vi "Test.Maui 2.0.Initialize.Plenty.Subpanels.Subpanel 1.vi"(8 "error in":errorcluster) -> (0 "error out":errorcluster)   [LabVIEW 2020]
uses:
  Maui 2.0/Maui 2.0.lvclass
  C:/Program Files (x86)/National Instruments/LabVIEW 2020/vi.lib/JKI/JKI SMO/SMO/SMO.lvclass
  Helper/Test Helper 1/Test Helper 1.lvclass
  <vilib>/addons/_JKI Toolkits/Caraya/classes/Assert/Assert Equal Value_Variant.vi
  <vilib>/JKI/JKI SMO/SMO/SMO.lvclass
  <vilib>/addons/_JKI Toolkits/Caraya/classes/Test/Test.lvclass
  <vilib>/addons/_JKI Toolkits/Caraya/classes/Assert/Assert.lvclass
panel:
  in  "Ring 2":u16(ring) items=["Test Helper 1", "Test Helper 1", "Maui 2.0", "None"]
  in  "Ring":u16(ring) items=["Test Helper 1", "Test Helper 1", "Maui 2.0", "None"]
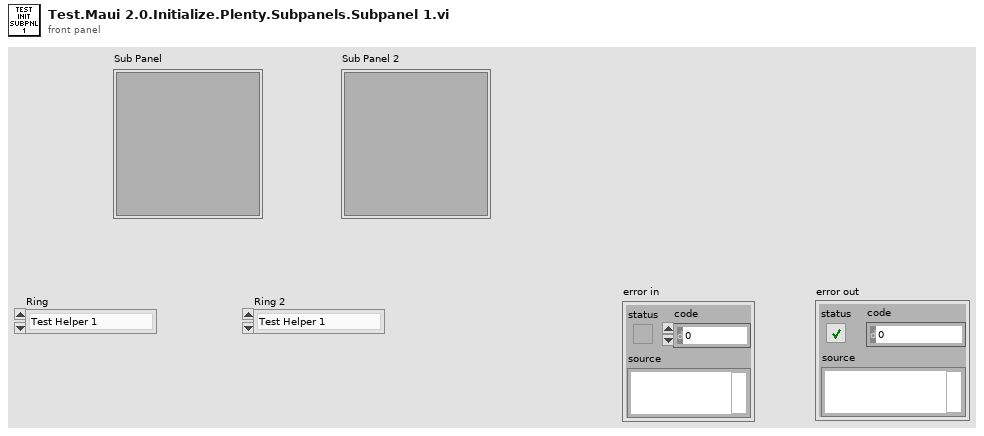
[diagram p1: front panel]
types:
  T1 = cluster{"Ring":refnum<vi>, "Sub Panel":refnum<vi>}
  T2 = cluster{"Ring 2":refnum<vi>, "Sub Panel 2":refnum<vi>}
  T3 = cluster{"Ring 2":refnum<vi>, "Sub Panel 2":refnum<vi>}[]
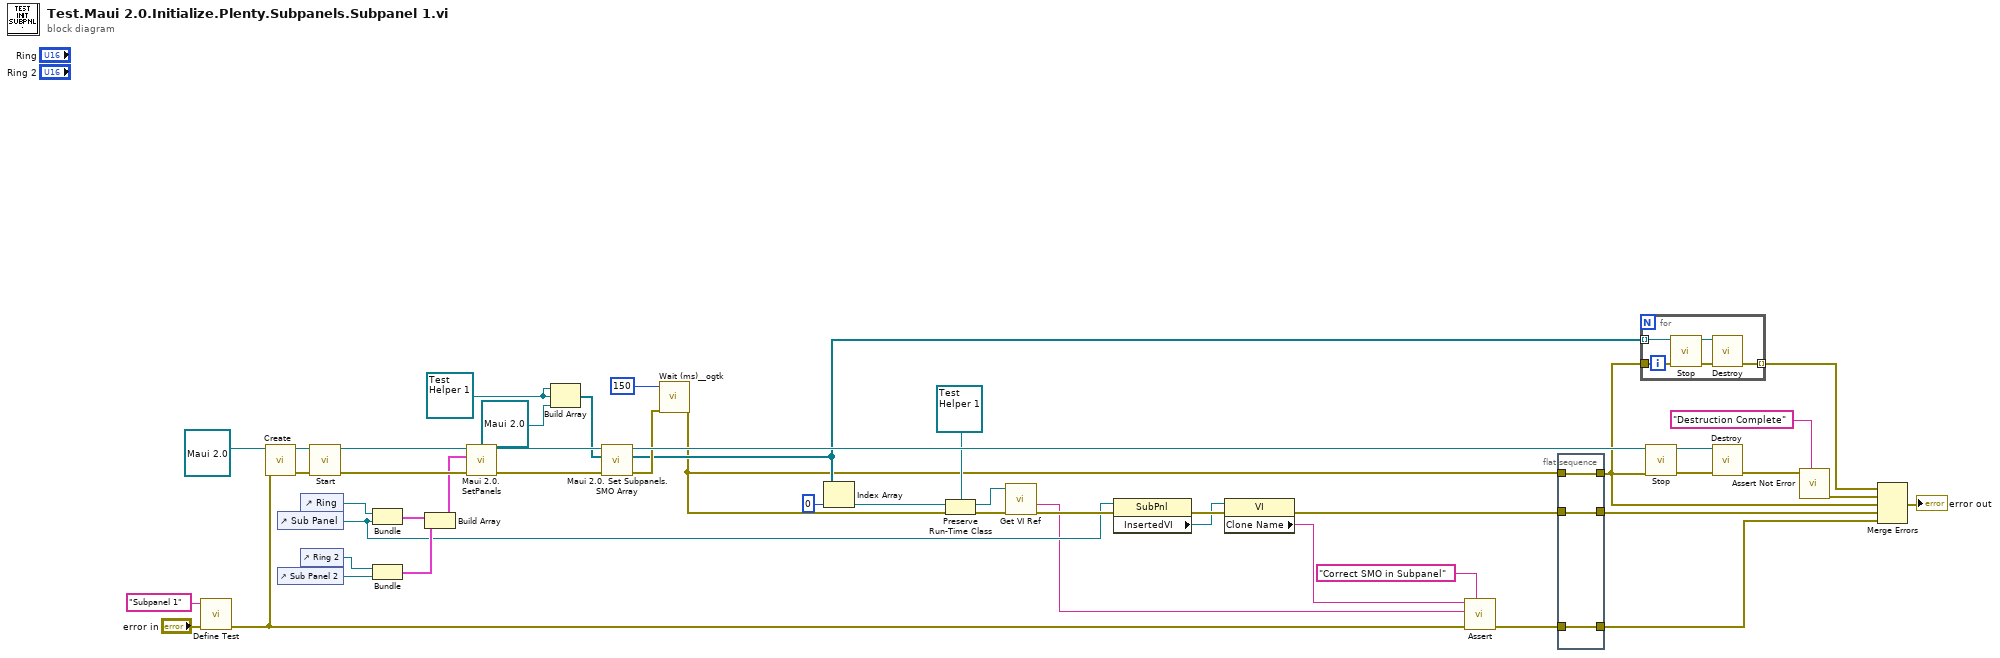
[diagram p0: block diagram]
diagram:
  w17 = refnum<class "Test Helper 1.lvclass"> refnum ("Test Helper 1.lvclass")
  n1 = call <vilib>:"Define Test.vi"("error in (no error)"="error in", "Label (VI Title)"="Subpanel 1") -> ("error out"=w20:errorcluster)  [unwired: 9 in]
  n2 = call <vilib>:"Create.vi"("error in (no error)"=w20, "SMO"=refnum<class "Maui 2.0.lvclass"> refnum ("Maui 2.0 in")) -> ("error out"=w48:errorcluster, "SMO out"=w41:refnum<class "Maui 2.0.lvclass">)  [unwired: 7 in, 1 out]
  n3 = control-ref of="Sub Panel"() -> (w9:refnum<vi>)
  n4 = control-ref of="Sub Panel 2"() -> (w44:refnum<vi>)
  n5 = control-ref of="Ring"() -> (w34:refnum<vi>)
  n6 = control-ref of="Ring 2"() -> (w45:refnum<vi>)
  n7 = call <vilib>:"Start.vi"("error in (no error)"=w48, "SMO"=w41) -> ("error out"=w47:errorcluster, "SMO out"=w39:refnum<class "Maui 2.0.lvclass">)  [unwired: 8 in]
  n8 = Bundle("Ring"=w34, "Sub Panel"=w9) -> (w43:T1)  [unwired: 1 in]
  n9 = Bundle("Ring 2"=w45, "Sub Panel 2"=w44) -> (w42:T2)  [unwired: 1 in]
  n10 = Build Array(w43, w42) -> (w35:T3)
  n11 = call "Maui 2.0.SetPanels.vi"("error in (no error)"=w47, "Set Panels"=w35, "Maui 2.0"=w39) -> ("error out"=w46:errorcluster, "Maui 2.0 out"=w38:refnum<class "Maui 2.0.lvclass">)  [unwired: 7 in]
  n12 = Build Array(w17, w17, refnum<class "Maui 2.0.lvclass"> refnum ("Maui 2.0 in")) -> (w36:refnum<class "SMO.lvclass">[])
  n13 = call-dynamic "Maui 2.0. Set Subpanels.SMO Array.vi"("error in (no error)"=w46, "Subpanels in"=w36, "Maui 2.0 in"=w38) -> ("error out"=w23:errorcluster, "Subpanels Out"=w5:refnum<class "SMO.lvclass">[], "Maui 2.0 out"=w31:refnum<class "Maui 2.0.lvclass">)  [unwired: 6 in]
  n14 = call <userlib>:"Wait (ms)__ogtk.vi"("error in (no error)"=w23, "milliseconds to wait"=u32 150) -> ("error out"=w4:errorcluster)  [unwired: 8 in, 1 out]
  n15 = Index Array(array=w5, index=0) -> (element=w19:refnum<class "SMO.lvclass">)
  n16 = Preserve Run-Time Class(object in=w19, error in=w4, 2:refnum<class "Test Helper 1.lvclass"> refnum ("Test Helper 1.lvclass")) -> (object out=w16:refnum<class "Test Helper 1.lvclass">, error out=w15:errorcluster)
  n17 = call-dynamic "Get VI Ref.vi"("error in (no error)"=w15, "Test Helper 1 in"=w16) -> ("error out"=w14:errorcluster, "VI Clone Name"=w3:string)  [unwired: 6 in, 2 out]
  n18 = property on="Property Node" class="SubPnl"(reference=w9, error in=w14) -> (error out=w12:errorcluster, "InsertedVI"=w10:refnum<vi>)  [unwired: 1 out]
  n19 = property on="Property Node" class="VI"(reference=w10, error in=w12) -> (error out=w11:errorcluster, "Clone Name"=w7:string)  [unwired: 1 out]
  n20 = call-poly <vilib>:"Assert.vi"("Label"="Correct SMO in Subpanel", "error in (no error)"=w20, "Y"=w3, "X"=w7) -> ("error out"=w8:errorcluster)  [unwired: 7 in]
  n21 = flat-sequence {
    tunnel: w4 -> [w51]
    tunnel: w11 -> [w50]
    tunnel: w8 -> [w49]
    tunnel: [w51] -> w21
    tunnel: [w50] -> w25
    tunnel: [w49] -> w24
    frame #0 {
    }
  }
  n22 = for {
    tunnel: w5 -> [w55] mode=indexing
    tunnel: w21 -> [w54]
    tunnel: [w52] -> w22 mode=indexing
    n23 = call <vilib>:"Stop.vi"("error in (no error)"=w54, "SMO"=w55) -> ("error out"=w53:errorcluster, "SMO out"=w56:refnum<class "SMO.lvclass">)  [unwired: 8 in]
    n24 = call <vilib>:"Destroy.vi"("error in (no error)"=w53, "SMO"=w56) -> ("error out"=w52:errorcluster)  [unwired: 9 in]
  }
  n25 = call <vilib>:"Stop.vi"("error in (no error)"=w21, "SMO"=w31) -> ("error out"=w29:errorcluster, "SMO out"=w30:refnum<class "Maui 2.0.lvclass">)  [unwired: 8 in]
  n26 = call <vilib>:"Destroy.vi"("error in (no error)"=w29, "SMO"=w30) -> ("error out"=w28:errorcluster)  [unwired: 9 in]
  n27 = call <vilib>:"Assert Not Error.vi"("Label"="Destruction Complete", "Not Error?"=w28) -> ("error out"=w26:errorcluster)  [unwired: 9 in]
  n28 = Merge Errors(w22, w26, w21, w25, w24) -> (→"error out":errorcluster)
